vi "create_ramp.vi"(1 "final value":dbl=1.0 format="%_6g", 2 "increment":dbl=1.0 format="%_6g", 3 "starting value":dbl format="%_6g") -> (0 "ramp data":dbl[](array[numeric]) format="%_6g")   [LabVIEW 2012]
panel:
  out "data count":i32
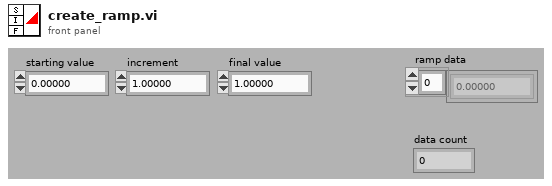
[diagram p1: front panel]
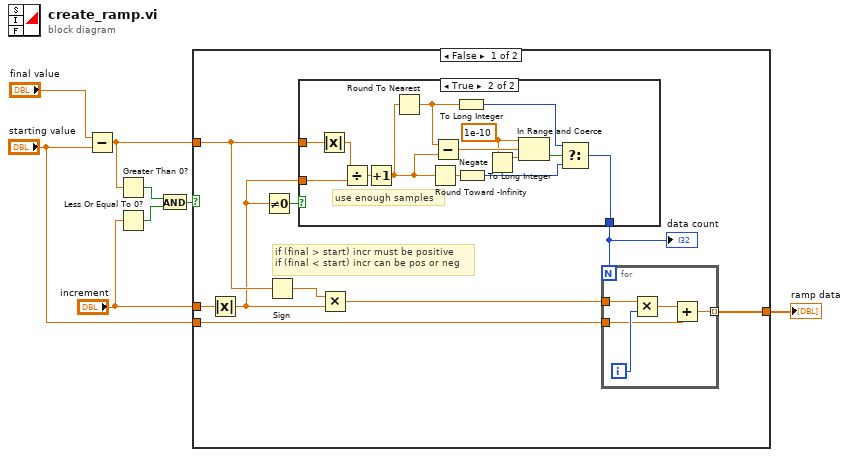
[diagram p0: block diagram]
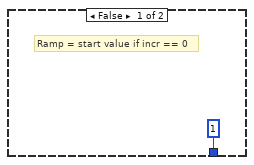
[diagram p2: hidden frame]
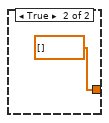
[diagram p3: hidden frame]
diagram:
  n1 = Subtract(x="final value", y="starting value") -> (x-y=w2:dbl)
  n2 = Greater Than 0?(x=w2) -> (x > 0?=w3:bool)
  n3 = Less Or Equal To 0?(x="increment") -> (x <= 0?=w4:bool)
  n4 = And(x=w3, y=w4) -> (x .and. y?=w1:bool)
  n5 = case shown="False" w1 {
    tunnel: "starting value" -> [w9 _]
    tunnel: [w11 dbl[] []] -> w6
    tunnel: "increment" -> [w15 _]
    tunnel: w2 -> [w17 _]
    frame False {
      # "if (final > start) incr must be positive\nif (final < start) incr can be pos or neg"
      n6 = Absolute Value(x=w15) -> (abs(x)=w13:dbl)
      n7 = Not Equal To 0?(x=w13) -> (x != 0?=w14:bool)
      n8 = Sign(1:w17) -> (0:w16:dbl)
      n9 = case shown="True" w14 {
        tunnel: [1 w23] -> w12
        tunnel: w17 -> [_ w20]
        tunnel: w13 -> [_ w19]
        frame False {
          # "Ramp = start value if incr == 0"
        }
        frame True {
          w29 = 1e-10 ("upper limit")
          # "use enough samples"
          n10 = Absolute Value(x=w20) -> (abs(x)=w21:dbl)
          n11 = Divide(x=w21, y=w19) -> (x/y=w22:dbl)
          n12 = Increment(x=w22) -> (x+1=w31:dbl)
          n13 = Round To Nearest(number=w31) -> (nearest integer value=w27:dbl)
          n14 = Round Toward -Infinity(1:w31) -> (0:w32:dbl)
          n15 = Subtract(x=w27, y=w31) -> (x-y=w30:dbl)
          n16 = To Long Integer(number=w27) -> (32bit integer=w26:i32)
          n17 = To Long Integer(number=w32) -> (32bit integer=w25:i32)
          n18 = Negate(x=w29) -> (-x=w24:dbl)
          n19 = In Range and Coerce(upper limit=w29, x=w30, lower limit=w24) -> (In Range?=w28:bool)  [unwired: 1 out]
          n20 = Select(t=w26, s=w28, f=w25) -> (s? t:f=w23:i32)
        }
      }
      "data count" <- w12
      n21 = Multiply(x=w16, y=w13) -> (x*y=w10:dbl)
      n22 = for {
        N: w12 -> [_]
        tunnel: [w37] -> w11 mode=indexing
        tunnel: w10 -> [w35]
        tunnel: w9 -> [w33]
        i -> [w36]
        n23 = Multiply(x=w35, y=w36) -> (x*y=w34:dbl)
        n24 = Add(x=w34, y=w33) -> (x+y=w37:dbl)
      }
    }
    frame True {
    }
  }
  "ramp data" <- w6
